vi "Get Actual Status.vi"(0 "COM Port in":refnum<visa-resource-name>, 1 "error in":errorcluster) -> (2 "COM Port out":refnum<visa-resource-name>, 3 "Actual Status":bool[](array[boolean]), 4 "OK":bool, 5 "error out":errorcluster)   [LabVIEW 2013]
doc: "This command gives back the actual operating status of the laser/led."
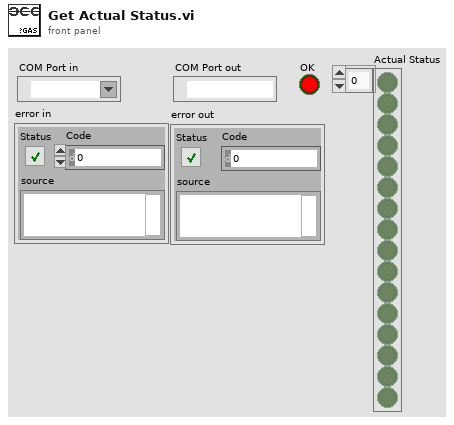
[diagram p1: front panel]
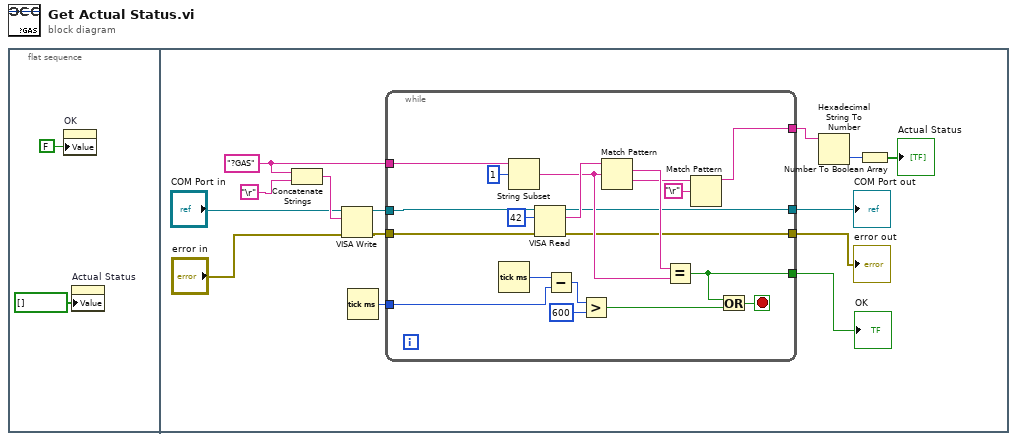
[diagram p0: block diagram]
diagram:
  n1 = flat-sequence {
    frame #0 {
      n2 = property on="OK" class="Bool. (strikt)"("Value"=FALSE ("OK")) -> ()  [unwired: 2 in, 2 out]
      n3 = property on="Actual Status" class="Arr (strikt)"("Value"=bool[] [] ("Actual Status")) -> ()  [unwired: 2 in, 2 out]
    }
    frame #1 {
      w7 = "?GAS" ("Schreibpuffer")
      n4 = Concatenate Strings(w7, "\r") -> (w13:string)
      n5 = VISA Write(VISA resource name="COM Port in", write buffer=w13, error in (no error)="error in") -> (VISA resource name out=w9:refnum<visa-resource-name>, error out=w8:errorcluster)  [unwired: 1 out]
      n6 = Tick Count (ms)() -> (millisecond timer value=w6:u32)
      n7 = while {
        tunnel: [w31] -> w16
        tunnel: [w30] -> w15
        tunnel: [w29] -> w5
        tunnel: [w25] -> w14
        tunnel: w9 -> [w18]
        tunnel: w8 -> [w27]
        tunnel: w7 -> [w26]
        tunnel: w6 -> [w22]
        stop <- w24 stop-if-true
        n8 = Tick Count (ms)() -> (millisecond timer value=w23:u32)
        n9 = String Subset(string=w26, offset (0)=1 ("Offset (0)")) -> (substring=w32:string)  [unwired: 1 in]
        n10 = VISA Read(VISA resource name=w18, byte count=u32 42 ("Byte-Anzahl"), error in (no error)=w27) -> (VISA resource name out=w31:refnum<visa-resource-name>, read buffer=w35:string, error out=w30:errorcluster)  [unwired: 1 out]
        n11 = Subtract(x=w23, y=w22) -> (x-y=w21:u32)
        n12 = Greater?(x=w21, y=u32 600) -> (0:w19:bool)
        n13 = Match Pattern(string=w35, regular expression=w32) -> (match substring=w34:string, after substring=w28:string)  [unwired: 1 in, 2 out]
        n14 = Equal?(x=w34, y=w32) -> (x = y?=w25:bool)
        n15 = Match Pattern(string=w28, regular expression="\r") -> (before substring=w29:string)  [unwired: 1 in, 3 out]
        n16 = Or(x=w25, y=w19) -> (x .or. y?=w24:bool)
      }
      "COM Port out" <- w16
      "error out" <- w15
      "OK" <- w14
      n17 = Hexadecimal String To Number(string=w5) -> (number=w4:u32)  [unwired: 2 in, 1 out]
      n18 = Number To Boolean Array(number=w4) -> (Boolean array=→"Actual Status":bool[])
    }
  }
